vi "rqcBob Cascade sync ui (Low Level Example).vi"() -> ()   [LabVIEW 2019]
uses:
  <vilib>/FTP/NI_FTP.lvlib
panel:
  out "cascade executed":bool=TRUE
  in  "local Corrected Bob's key path":path
  out "receiving Alice's picture":bool=TRUE
  out "Bob's key received":bool=TRUE
  in  "start receiving Alice's picture":bool
  in  "QBER":dbl
  in  "local Raw Bob's key path":path=path "../python_scripts/cascade_alice.py"
  out "picture demo script path":path=path "../python_scripts/cascade_alice.py"
  out "remote BobKey.bin path":string
  out "Alices's user password":string
  out "Alices's user login":string
  in  "error in":errorcluster
  in  "FTP request bob's key":bool
  in  "cascade switch":bool
  in  "stop":bool
  in  "Alices's port":string
  in  "Alices's IP":string
  out "?":T1
  out "?":picture
  out "cascade script path":path=path "../python_scripts/cascade_alice.py"
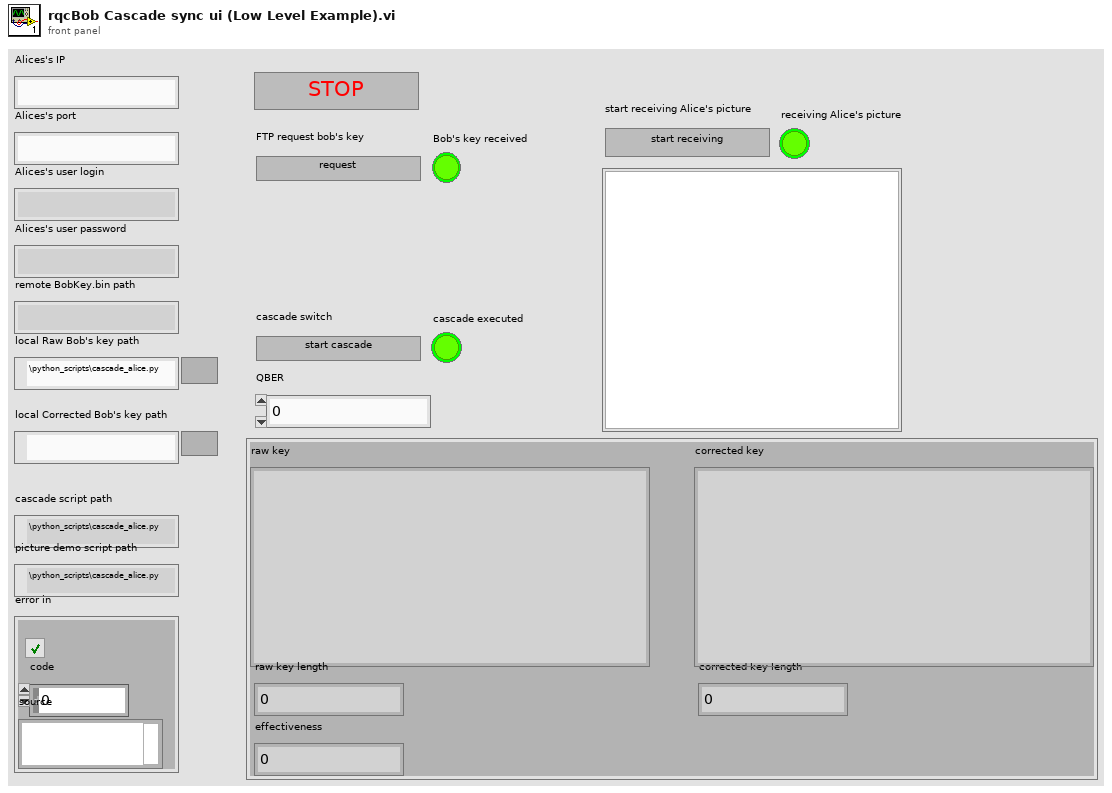
[diagram p1: front panel]
types:
  T1 = cluster{"raw key length":i32, "corrected key":string, "corrected key length":i32, "effectiveness":dbl, "raw key":string}
  T2 = typedef "imagedata.ctl" = cluster{"image type":i32, "image depth":i32, "image":u8[], "mask":u8[], "colors":u32[], "Rectangle":cluster{"left":i16, "top":i16, "right":i16, "bottom":i16}}
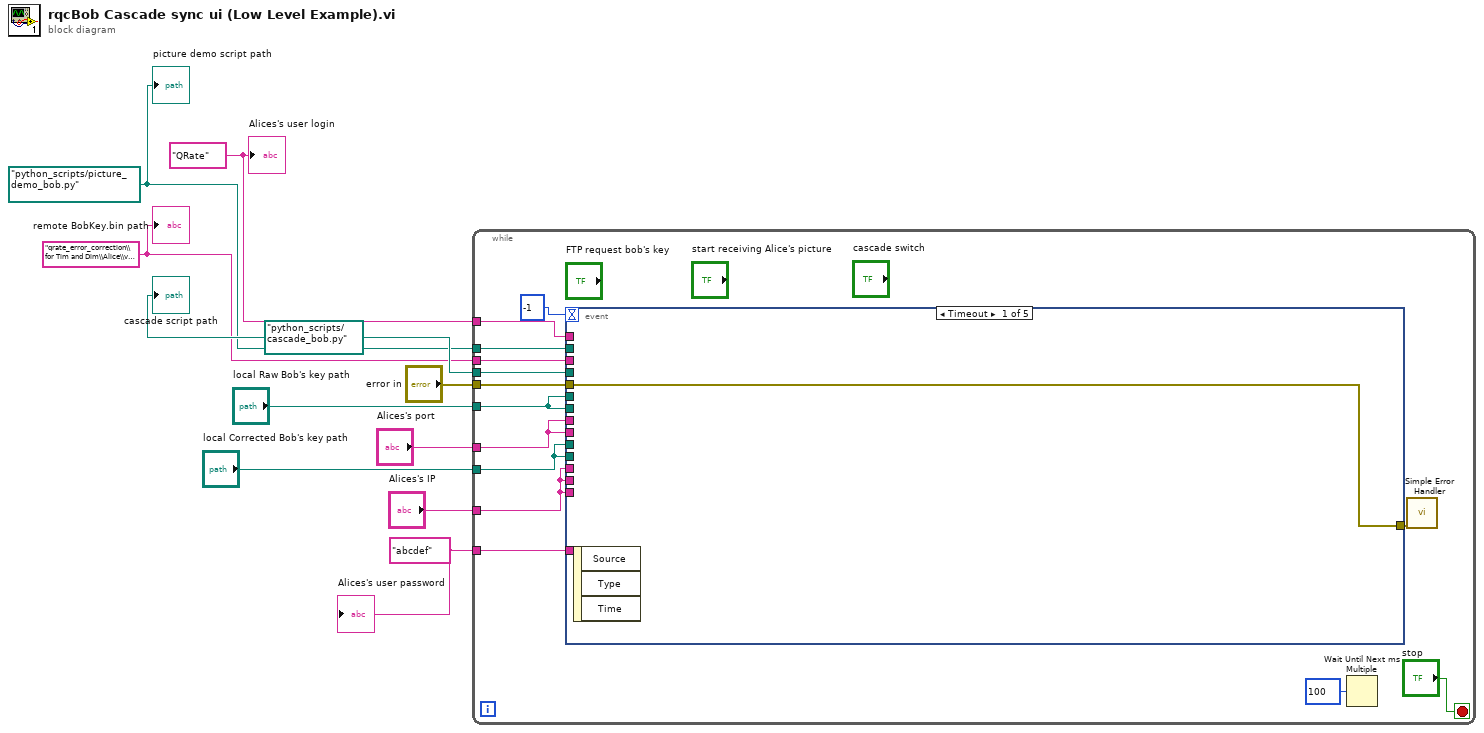
[diagram p0: block diagram]
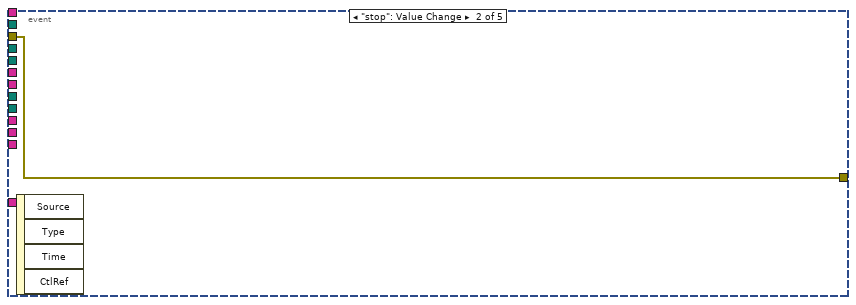
[diagram p2: hidden frame]
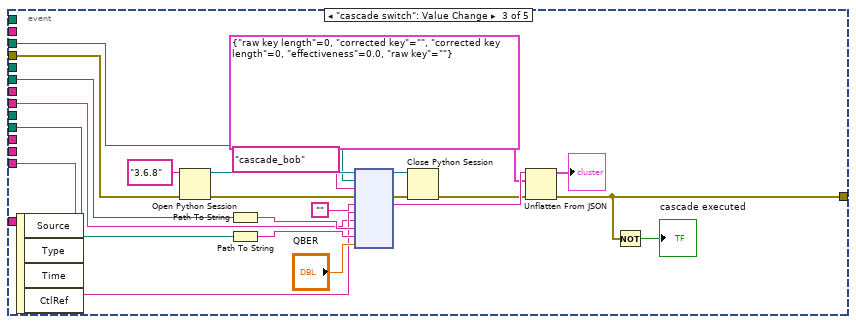
[diagram p3: hidden frame]
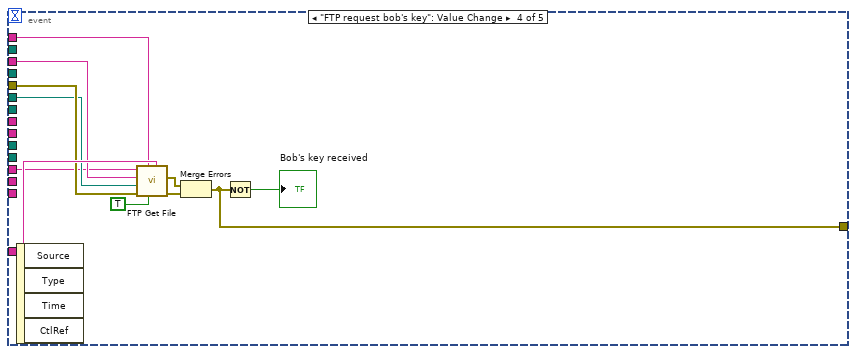
[diagram p4: hidden frame]
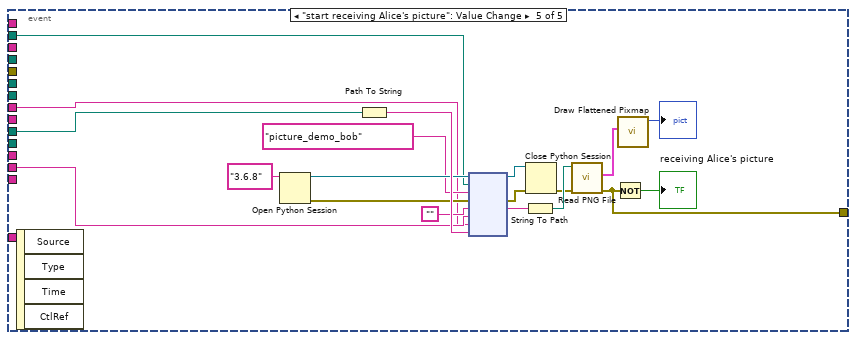
[diagram p5: hidden frame]
diagram:
  w3 = path "python_scripts/picture_demo_bob.py" ("module path")
  w4 = "qrate_error_correction\\for Tim and Dim\\Alice\\v 2.3.0 NewWave\\Host\\Alice Host Library\\Examples\\Low Level\\BobKey.bin" ("Alices's port 3")
  w6 = "abcdef" ("Alices's port 3")
  w5 = "QRate" ("Alices's port 3")
  w7 = path "python_scripts/cascade_bob.py"
  n1 = while {
    tunnel: "error in" -> [w19]
    tunnel: "Alices's port" -> [w13]
    tunnel: "Alices's IP" -> [w14]
    tunnel: w7 -> [w23]
    tunnel: w6 -> [w21]
    tunnel: w5 -> [w20]
    tunnel: w4 -> [w17]
    tunnel: w3 -> [w15]
    tunnel: "local Raw Bob's key path" -> [w18]
    tunnel: "local Corrected Bob's key path" -> [w16]
    stop <- "stop" stop-if-true
    n2 = event shown="[0] Timeout" {
      selector: _ -> [_ _ _ _ _]
      dyn-events: _ -> [_ _ _ _ _]
      timeout: -1 -> [_ _ _ _ _]
      tunnel: w16 -> [_ _ w38 _ _]
      tunnel: w18 -> [_ _ w37 _ _]
      tunnel: w23 -> [_ _ w34 _ _]
      tunnel: w14 -> [_ _ w31 _ _]
      tunnel: w13 -> [_ _ w30 _ _]
      tunnel: w21 -> [_ _ _ w56 _]
      tunnel: w20 -> [_ _ _ w54 _]
      tunnel: w19 -> [w25 w26 w28 w53 _]
      tunnel: w18 -> [_ _ _ w52 _]
      tunnel: w17 -> [_ _ _ w51 _]
      tunnel: w14 -> [_ _ _ w50 _]
      tunnel: w16 -> [_ _ _ _ w67]
      tunnel: w15 -> [_ _ _ _ w65]
      tunnel: w14 -> [_ _ _ _ w62]
      tunnel: w13 -> [_ _ _ _ w61]
      tunnel: [w25 w26 w27 w49 w60] -> w12
      event Timeout {
        n3 = event-data() -> ()  [unwired: 1 in, 3 out]
      }
      event "stop": Value Change {
        n4 = event-data() -> ()  [unwired: 1 in, 4 out]
      }
      event "cascade switch": Value Change {
        n5 = event-data() -> ()  [unwired: 1 in, 4 out]
        n6 = Open Python Session(python version="3.6.8" ("Python version"), 3:w28) -> (session out=w39:refnum<k35>, error out=w40:errorcluster)  [unwired: 1 in]
        n7 = Path To String(path=w37) -> (string=w43:string)
        n8 = Path To String(path=w38) -> (string=w45:string)
        n9 = node(w39, w34, "cascade_bob" ("function name"), w40, "", w31, w30, w43, w45, "QBER") -> (w41:refnum<k35>, w42:errorcluster, w47:string)  [unwired: 5 in, 2 out]
        n10 = Close Python Session(session in=w41, error in=w42) -> (11:w46:errorcluster)
        n11 = Unflatten From JSON(JSON string=w47, type and defaults=T1 {"raw key length"=0, "corrected key"="", "corrected key length"=0, "effectiveness"=0.0, "raw key"=""}, error in (no error)=w46) -> (value=→"?":T1, error out=w27:errorcluster)  [unwired: 4 in]
        n12 = Not(x=w27) -> (.not. x?=→"cascade executed":bool)
      }
      event "FTP request bob's key": Value Change {
        n13 = event-data() -> ()  [unwired: 1 in, 4 out]
        n14 = call <vilib>:"FTP Get File.vi"("password"=w56, "binary (F)"=TRUE, "user"=w54, "error in (no error)"=w53, "local path"=w52, "remote path"=w51, "host"=w50) -> ("error out"=w57:errorcluster, "file error"=w58:errorcluster)  [unwired: 3 in]
        n15 = Merge Errors(w58, w57) -> (w49:errorcluster)
        n16 = Not(x=w49) -> (.not. x?=→"Bob's key received":bool)
      }
      event "start receiving Alice's picture": Value Change {
        n17 = event-data() -> ()  [unwired: 1 in, 4 out]
        n18 = Open Python Session(python version="3.6.8" ("Python version")) -> (session out=w72:refnum<k35>, error out=w73:errorcluster)  [unwired: 2 in]
        n19 = Path To String(path=w67) -> (string=w78:string)
        n20 = node(w72, w65, "picture_demo_bob" ("function name"), w73, "", w62, w61, w78) -> (w74:refnum<k35>, w75:errorcluster, w76:string)  [unwired: 3 in, 2 out]
        n21 = String To Path(string=w76) -> (path=w77:path)
        n22 = Close Python Session(session in=w74, error in=w75) -> (11:w69:errorcluster)
        n23 = call <vilib>:"Read PNG File.vi"("error in (no error)"=w69, "path to PNG file"=w77) -> ("error out"=w60:errorcluster, "image data"=w70:T2)  [unwired: 7 in, 1 out]
        n24 = Not(x=w60) -> (.not. x?=→"receiving Alice's picture":bool)
        n25 = call <vilib>:"Draw Flattened Pixmap.vi"("image data"=w70) -> ("new picture"=→"?":picture)  [unwired: 8 in]
      }
    }
    n26 = Wait Until Next ms Multiple(millisecond multiple=u32 100) -> ()  [unwired: 1 out]
    n27 = call <vilib>:"Simple Error Handler.vi"("error in (no error)"=w12) -> ()  [unwired: 4 in, 5 out]
  }
  "cascade script path" <- w7
  "Alices's user login" <- w5
  "Alices's user password" <- w6
  "remote BobKey.bin path" <- w4
  "picture demo script path" <- w3
